vi "WPI_UtilitiesFRCAutomaticValuePublisher.vi"   [LabVIEW 2017]
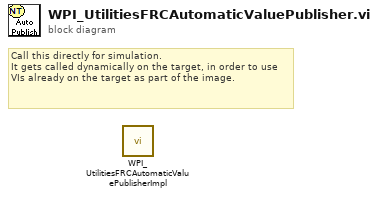
[diagram p0: block diagram]
diagram:
  # "Call this directly for simulation.\nIt gets called dynamically on the target, in order to use VIs already on the target as part of the image."
  n1 = call <vilib>:"WPI_UtilitiesFRCAutomaticValuePublisherImpl.vi"() -> ()  [unwired: 12 in]
